vi "Draw.vi"(8 "Error In":errorcluster, 11 "Pixel In":refnum<class "Pixel.lvclass">) -> (0 "Error Out":errorcluster, 2 "Element To Display":T1[](array[typedef]), 3 "Pixel Out":refnum<class "Pixel.lvclass">)   [LabVIEW 2019, in "Pixel.lvclass"]
uses:
  Pixel.lvclass
  C:/Users/goo13/Documents/GIT Local/myRIO-Neopixel/Source/RT/Display Element/Display Element.lvclass
  Display Element/Public/Controls/Pixel.ctl
  Display Utilities/Public/Controls/2D Coordinates.ctl
  Display Utilities/Display Utilities.lvlib
  Display Element/Display Element.lvclass
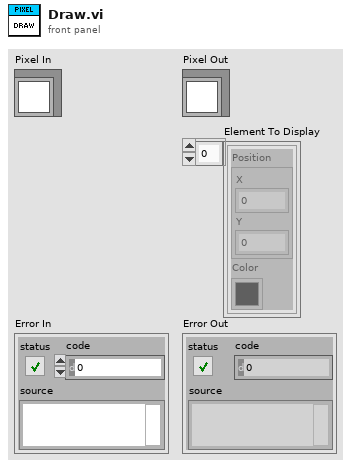
[diagram p1: front panel]
types:
  T1 = typedef "Display Element.lvclass/Pixel.ctl" = cluster{"Position":T2, "Color":u32}
  T2 = typedef "Display Utilities.lvlib/2D Coordinates.ctl" = cluster{"X":i32, "Y":i32}
  T3 = typedef "Display Element.lvclass/Vector.ctl" = cluster{"X":i32, "Y":i32}
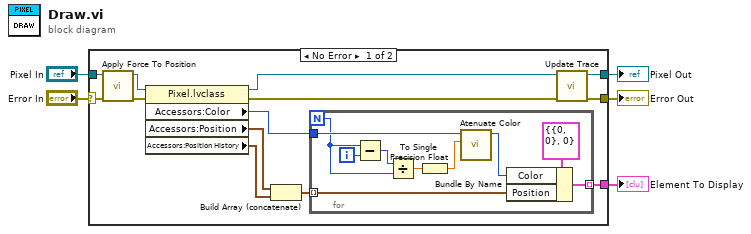
[diagram p0: block diagram]
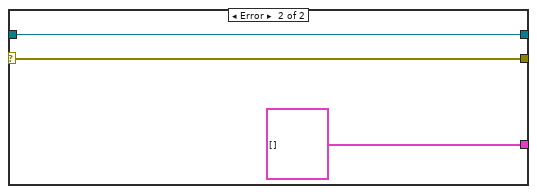
[diagram p2: hidden frame]
diagram:
  n1 = case shown="No Error" "Error In" {
    selector: "Error In" -> [w10 w31]
    tunnel: "Pixel In" -> [w9 w30]
    tunnel: [w15 w31] -> w3
    tunnel: [w16 w30] -> w2
    tunnel: [w11 T1[] []] -> w1
    frame No Error {
      n2 = call-dynamic "Apply Force To Position.vi"("Error In"=w10, "Display Element In"=w9) -> ("Error Out"=w8:errorcluster, "Display Element Out"=w7:refnum<class "Pixel.lvclass">)  [unwired: 8 in]
      n3 = property class="Pixel.lvclass"(reference=w7, error in=w8) -> (reference out=w18:refnum<class "Pixel.lvclass">, error out=w17:errorcluster, "Accessors:Color"=w12:u32, "Accessors:Position"=w14:T3, "Accessors:Position History"=w6:T3[])
      n4 = Build Array (concatenate)(w14, w6) -> (w13:T3[])
      n5 = for {
        N -> [w21]
        tunnel: w13 -> [w27] mode=indexing
        tunnel: w12 -> [w24]
        tunnel: [w26] -> w11 mode=indexing
        i -> [w23]
        n6 = Subtract(x=w21, y=w23) -> (x-y=w22:i32)
        n7 = Divide(x=w22, y=w21) -> (x/y=w20:dbl)
        n8 = To Single Precision Float(number=w20) -> (single precision float=w19:sgl)
        n9 = call "Atenuate Color.vi"("Gain"=w19, "Color In"=w24) -> ("Color Out"=w25:u32)  [unwired: 9 in]
        n10 = Bundle By Name(cluster=T1 {"Position"={"X"=0, "Y"=0}, "Color"=0} ("Pixel"), "Color"=w25, "Position"=w27) -> (w26:T1)
      }
      n11 = call "Update Trace.vi"("Error In"=w17, "Pixel In"=w18) -> ("Error Out"=w15:errorcluster, "Pixel Out"=w16:refnum<class "Pixel.lvclass">)  [unwired: 8 in]
    }
    frame Error {
    }
  }
  "Pixel Out" <- w2
  "Error Out" <- w3
  "Element To Display" <- w1
